vi "Get Error Line Format.vi"(8 "error in (no error)":errorcluster, 11 "HSE_v2_Formatter in":refnum<class "HSE_v2_Formatter.lvclass">) -> (0 "error out":errorcluster, 2 "Error Line Format":string, 3 "HSE_v2_Formatter out":refnum<class "HSE_v2_Formatter.lvclass">)   [LabVIEW 2024, in "hse-logger.lvlib" / "HSE_v2_Formatter.lvclass"]
doc: "____\nHAMPEL SOFTWARE ENGINEERING v2.2.2 (2025-01-16 15:41)"
uses:
  <vilib>/Hampel Software Engineering/HSE Logger/Formatter/HSE_v2_Formatter/HSE_v2_Formatter.lvclass
  <vilib>/Hampel Software Engineering/HSE Logger/Formatter/HSE_v2_Formatter/HSE_v2_Formatter.lvclass/HSE_v2_Formatter.ctl
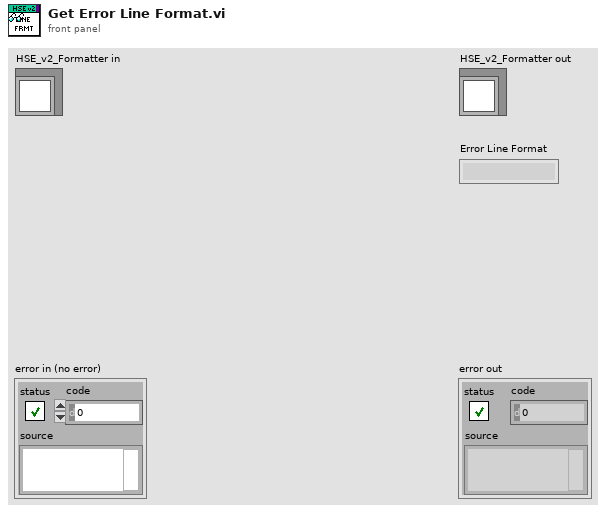
[diagram p1: front panel]
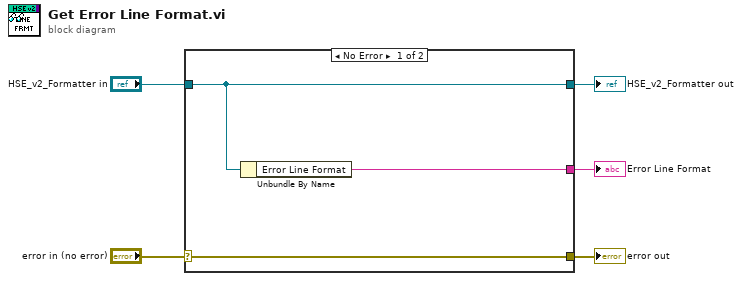
[diagram p0: block diagram]
diagram:
  n1 = case shown="No Error" "error in (no error)" {
    selector: "error in (no error)" -> [w8 w9]
    tunnel: [w8 w9] -> w4
    tunnel: [w7 w10] -> w2
    tunnel: "HSE_v2_Formatter in" -> [w7 w10]
    tunnel: [w6 _] -> w1
    frame No Error {
      n2 = Unbundle By Name(w7) -> ("Error Line Format"=w6:string)
    }
    frame Error {
    }
  }
  "error out" <- w4
  "HSE_v2_Formatter out" <- w2
  "Error Line Format" <- w1
